vi "Call Functional Global Variable.vi"() -> ()   [LabVIEW 2012]
uses:
  Resources/Action Items.ctl
panel:
  out "Result":i32
  in  "Initialize to":i32
  in  "Action":T1
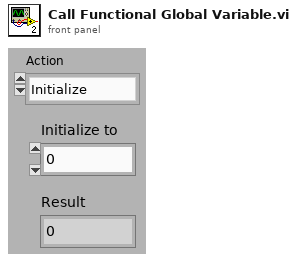
[diagram p1: front panel]
types:
  T1 = typedef "Action Items.ctl" = enum16{"Initialize", "Get", "Increment"}
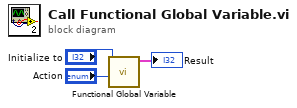
[diagram p0: block diagram]
diagram:
  n1 = call "Functional Global Variable.vi"("Action"="Action", "Mode"="Initialize to") -> ("Mode"=→"Result":cluster{"Run":bool, "Hold":bool, "Off":bool})  [unwired: 9 in]
